vi "温度警告.vi"() -> ()   [LabVIEW 2022 SP3]
panel:
  in  "温度下限":dbl
  out "低温警告":bool
  in  "温度上限":dbl
  out "波形图表":dbl(graph)
  out "高温警告":bool
  out "温度计":dbl(slide) scale=0.0..100.0
  in  "停止":bool
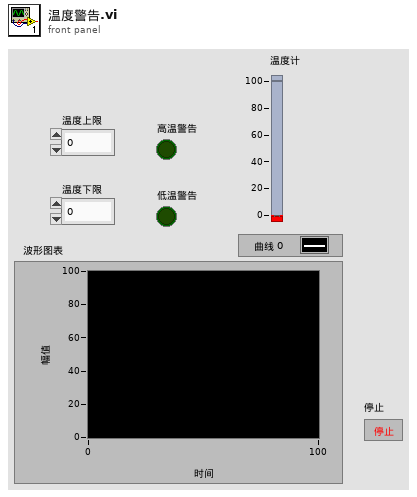
[diagram p1: front panel]
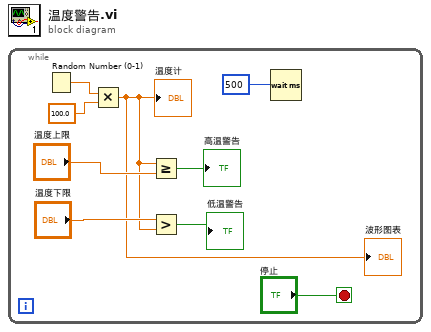
[diagram p0: block diagram]
diagram:
  n1 = while {
    stop <- "停止" stop-if-true
    n2 = Random Number (0-1)() -> (number: 0 to 1=w9:dbl)
    n3 = Multiply(x=w9, y=100.0) -> (x*y=w1:dbl)
    "温度计" <- w1
    "波形图表" <- w1
    n4 = Greater Or Equal?(x=w1, y="温度上限") -> (x >= y?=→"高温警告":bool)
    n5 = Greater?(x="温度下限", y=w1) -> (0:→"低温警告":bool)
    n6 = Wait (ms)(milliseconds to wait=500) -> ()  [unwired: 1 out]
  }
